vi "SVFA Wrap or Unwrap Phase (XY) (1 Ch).vi"(0 "phase spectrum in":cluster{"X":dbl[], "phase":dbl[]} {"phase" format="%.2f"; "X" format="%.2f"}, 1 "desired wrapping":T8(ring)=enum."Wrap: -180 to 180", 2 "custom wrap range":T1={"minimum phase"=-inf, "maximum phase"=inf}, 4 "spectrum info":T2={"channel name"="", "description"="", "x-axis units"=0, "spectral info"={"spectrum type"=enum."Power [Magnitude^2]", "linear/dB"=enum."linear", "window"=0, "window size"=0, "FFT size"=0}, "engineering units"=1, "custom label"="", "dB reference [EU]"=0.0, "peak units"=enum."rms", "weighting filter"=0, "spectral density?"=FALSE, "unit label"="", "spectrum skewed?"=FALSE, "complimentary spectrum units"=enum."none"} {"x-axis units" items=["Time (s)"=0, "Frequency-CB (Hz)"=1, "Frequency-CPB (Hz)"=1248, "Frequency-Arbitrary (Hz)"=2357, "Quefrency (s)"=2, "Revolutions (rev)"=3, "Order"=4, "Speed (RPM)"=11, "Speed (rad/s)"=21, "Index"=65535]; "weighting filter" items=["Linear", "A-weighting", "B-weighting", "C-weighting", "ITU-R 468-4", "Dolby", "CCITT", "C-message", "Wb", "Wc", "Wd", "We", "Wf", "Wh", "Wj", "Wk", "Wm", "AES17 20 kHz lowpass", "AES17 40 kHz lowpass", "AES17 20 kHz highpass", "AES17 40 kHz highpass"]; "dB reference [EU]" format="%.2f"; "engineering units" items=["custom..."=0, "V"=1, "A"=21, "C"=30, "pC"=31, "s"=32, "-"=29, "Pa"=2, "N"=20, "g"=3, "m/s^2"=4, "m/s"=5, "m"=6, "mm/s"=12, "mm"=13, "micron/s"=14, "micron"=15, "in/s^2"=7, "in/s"=8, "in"=9, "mil/s"=10, "mil"=11, "rad/s^2"=16, "rad/s"=17, "rad"=18, "deg/s^2"=26, "deg/s"=27, "deg"=28, "RPM"=22, "cycle/s^2"=23, "Hz"=24, "cycle"=25, "strain"=19]; "spectral info"."window" items=["None "=0, "Hanning"=1, "Hamming"=2, "Blackman-Harris"=3, "Exact Blackman"=4, "Blackman"=5, "Flat Top"=6, "4 Term B-Harris "=7, "7 Term B-Harris"=8, "Low Sidelobe"=9, "Force - Exponential"=10, "Gaussian"=62]}, 5 "error in (no error)":errorcluster) -> (14 "phase spectrum out":cluster{"X":dbl[], "phase":dbl[]} {"phase" format="%.2f"; "X" format="%.2f"}, 15 "unit label":string, 18 "dup spectrum info":T2={"channel name"="", "description"="", "x-axis units"=0, "spectral info"={"spectrum type"=enum."Power [Magnitude^2]", "linear/dB"=enum."linear", "window"=0, "window size"=0, "FFT size"=0}, "engineering units"=1, "custom label"="", "dB reference [EU]"=0.0, "peak units"=enum."rms", "weighting filter"=0, "spectral density?"=FALSE, "unit label"="", "spectrum skewed?"=FALSE, "complimentary spectrum units"=enum."none"} {"x-axis units" items=["Time (s)"=0, "Frequency-CB (Hz)"=1, "Frequency-CPB (Hz)"=1248, "Frequency-Arbitrary (Hz)"=2357, "Quefrency (s)"=2, "Revolutions (rev)"=3, "Order"=4, "Speed (RPM)"=11, "Speed (rad/s)"=21, "Index"=65535]; "weighting filter" items=["Linear", "A-weighting", "B-weighting", "C-weighting", "ITU-R 468-4", "Dolby", "CCITT", "C-message", "Wb", "Wc", "Wd", "We", "Wf", "Wh", "Wj", "Wk", "Wm", "AES17 20 kHz lowpass", "AES17 40 kHz lowpass", "AES17 20 kHz highpass", "AES17 40 kHz highpass"]; "dB reference [EU]" format="%.2f"; "engineering units" items=["custom..."=0, "V"=1, "A"=21, "C"=30, "pC"=31, "s"=32, "-"=29, "Pa"=2, "N"=20, "g"=3, "m/s^2"=4, "m/s"=5, "m"=6, "mm/s"=12, "mm"=13, "micron/s"=14, "micron"=15, "in/s^2"=7, "in/s"=8, "in"=9, "mil/s"=10, "mil"=11, "rad/s^2"=16, "rad/s"=17, "rad"=18, "deg/s^2"=26, "deg/s"=27, "deg"=28, "RPM"=22, "cycle/s^2"=23, "Hz"=24, "cycle"=25, "strain"=19]; "spectral info"."window" items=["None "=0, "Hanning"=1, "Hamming"=2, "Blackman-Harris"=3, "Exact Blackman"=4, "Blackman"=5, "Flat Top"=6, "4 Term B-Harris "=7, "7 Term B-Harris"=8, "Low Sidelobe"=9, "Force - Exponential"=10, "Gaussian"=62]}, 19 "error out":errorcluster)   [LabVIEW 2017]
doc: "Wraps the phase spectra to the specified range, so that all phase values are coerced to the specified band. You also can use this VI to unwrap phase spectra to eliminate discontinuities with absolute values exceeding 180 degrees = pi radians = 0.5 cycles. Wire data to the <B>phase spectrum in</B> input to determine the polymorphic instance to use or manually select the instance."
uses:
  <vilib>/addons/_NISVFA/_Shared subVIs/Controls/svc_Spectrum Info.ctl
  <vilib>/addons/_NISVFA/_Shared subVIs/Controls/svc_X-Axis Units.ctl
  <vilib>/addons/_NISVFA/_Shared subVIs/Controls/svc_Spectrum Type.ctl
  <vilib>/addons/_NISVFA/_Shared subVIs/Controls/svc_Engineering Units Text Ring.ctl
  <vilib>/addons/_NISVFA/_Shared subVIs/Controls/svc_Weighting Filter Text Ring.ctl
  <vilib>/addons/_NISVFA/_Shared subVIs/Controls/svc_Complimentary Spectrum Units.ctl
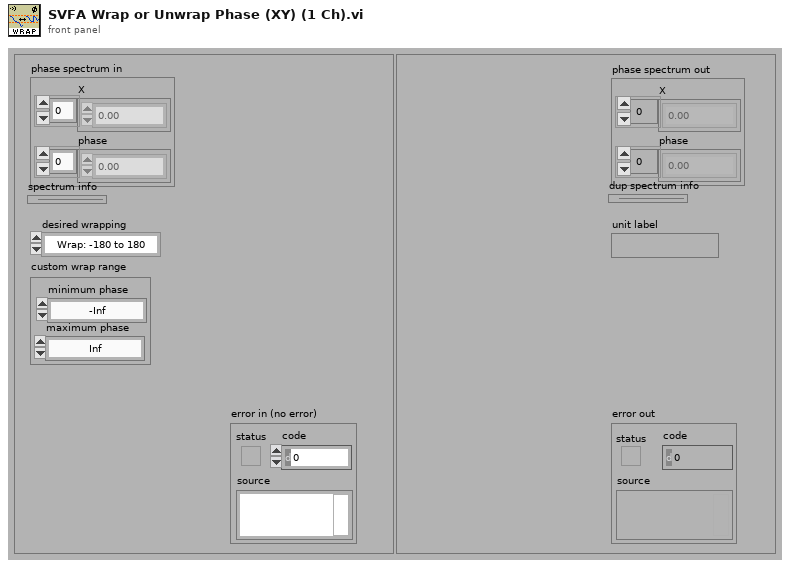
[diagram p1: front panel]
types:
  T1 = cluster{"minimum phase":dbl, "maximum phase":dbl}
  T2 = typedef "svc_Spectrum Info.ctl" = cluster{"channel name":string, "description":string, "x-axis units":T3, "spectral info":cluster{"spectrum type":T4, "linear/dB":enum16{"linear", "dB"}, "window":u16, "window size":i32, "FFT size":i32}, "engineering units":T5, "custom label":string, "dB reference [EU]":dbl, "peak units":enum16{"rms", "peak", "peak-peak"}, "weighting filter":T6, "spectral density?":bool, "unit label":string, "spectrum skewed?":bool, "complimentary spectrum units":T7}
  T3 = typedef "svc_X-Axis Units.ctl" = u16
  T4 = typedef "svc_Spectrum Type.ctl" = enum16{"FFT Spectrum [complex]", "Amplitude [Magnitude]", "Power [Magnitude^2]", "Cross Spectrum [complex]", "Frequency Response [Complex]"}
  T5 = typedef "svc_Engineering Units Text Ring.ctl" = u16
  T6 = typedef "svc_Weighting Filter Text Ring.ctl" = u16
  T7 = typedef "svc_Complimentary Spectrum Units.ctl" = enum16{"none", "radians", "degrees", "cycles", "imaginary"}
  T8 = enum16{"No change", "Unwrap", "Wrap: -360 to 0", "Wrap: -270 to 90", "Wrap: -180 to 180", "Wrap: -90 to 270", "Wrap: 0 to 360", "Wrap: custom range"}
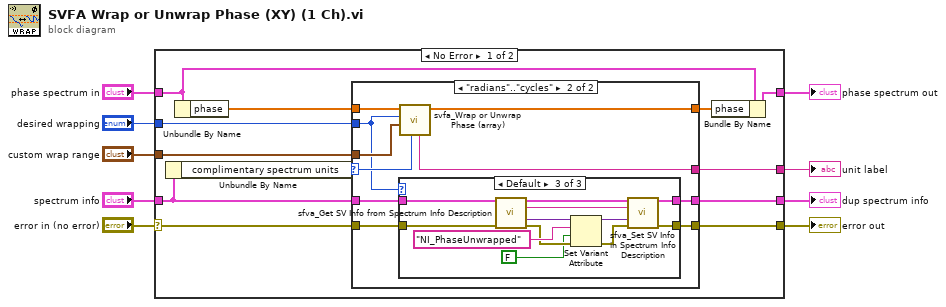
[diagram p0: block diagram]
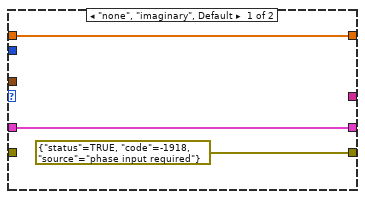
[diagram p2: hidden frame]
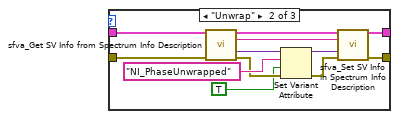
[diagram p4: hidden frame]
diagram:
  n1 = case shown="No Error" "error in (no error)" {
    selector: "error in (no error)" -> [w13 w62]
    tunnel: "phase spectrum in" -> [w16 w63]
    tunnel: [w15 w63] -> w8
    tunnel: [w12 w62] -> w2
    tunnel: "desired wrapping" -> [w18 _]
    tunnel: "spectrum info" -> [w11 w61]
    tunnel: [w10 w61] -> w3
    tunnel: [w19 _] -> w4
    tunnel: "custom wrap range" -> [w17 _]
    frame No Error {
      n2 = Unbundle By Name(w11) -> ("complimentary spectrum units"=w14:T7)
      n3 = Unbundle By Name(w16) -> ("phase"=w20:dbl[])
      n4 = case shown="\"radians\"..\"cycles\"" w14 {
        selector: w14 -> [_ w30]
        tunnel: [w24 w34] -> w21
        tunnel: w20 -> [w24 w33]
        tunnel: [_ w32] -> w19
        tunnel: w18 -> [_ w25]
        tunnel: w17 -> [_ w31]
        tunnel: w13 -> [_ w26]
        tunnel: [errorcluster {"status"=TRUE, "code"=-1918, "source"="phase input required"} ("error IO") w27] -> w12
        tunnel: w11 -> [w22 w29]
        tunnel: [w22 w28] -> w10
        frame "none", "imaginary", Default {
        }
        frame "radians".."cycles" {
          n5 = case shown="Default" w25 {
            tunnel: w29 -> [w36 w41 w53]
            tunnel: [w36 w40 w52] -> w28
            tunnel: [w35 w39 w51] -> w27
            tunnel: w26 -> [w35 w38 w50]
            frame "No change" {
            }
            frame "Unwrap" {
              n6 = call <vilib>:"sfva_Get SV Info from Spectrum Info Description.vi"("spectrum info"=w41, "error in (no error)"=w38) -> ("spectrum info"=w48:T2, "description"=w47:string, "SV Info"=w43:variant, "error out"=w42:errorcluster)  [unwired: 9 in, 1 out]
              n7 = Set Variant Attribute(Variant=w43, name="NI_PhaseUnwrapped", value=TRUE ("replaced"), error in=w42) -> (Variant out=w44:variant, error out=w45:errorcluster)  [unwired: 1 out]
              n8 = call <vilib>:"sfva_Set SV Info in Spectrum Info Description.vi"("spectrum info"=w48, "description"=w47, "SV Info"=w44, "error in (no error)"=w45) -> ("spectrum info"=w40:T2, "error out"=w39:errorcluster)  [unwired: 10 in]
            }
            frame Default {
              n9 = call <vilib>:"sfva_Get SV Info from Spectrum Info Description.vi"("spectrum info"=w53, "error in (no error)"=w50) -> ("spectrum info"=w60:T2, "description"=w59:string, "SV Info"=w55:variant, "error out"=w54:errorcluster)  [unwired: 9 in, 1 out]
              n10 = Set Variant Attribute(Variant=w55, name="NI_PhaseUnwrapped", value=FALSE ("replaced"), error in=w54) -> (Variant out=w56:variant, error out=w57:errorcluster)  [unwired: 1 out]
              n11 = call <vilib>:"sfva_Set SV Info in Spectrum Info Description.vi"("spectrum info"=w60, "description"=w59, "SV Info"=w56, "error in (no error)"=w57) -> ("spectrum info"=w52:T2, "error out"=w51:errorcluster)  [unwired: 10 in]
            }
          }
          n12 = call <vilib>:"svfa_Wrap or Unwrap Phase (array).vi"("phase units"=w30, "custom wrap range"=w31, "desired wrapping"=w25, "phase in"=w33) -> ("phase out"=w34:dbl[], "unit label"=w32:string)  [unwired: 6 in]
        }
      }
      n13 = Bundle By Name(cluster=w16, "phase"=w21) -> (w15:cluster{"X":dbl[], "phase":dbl[]})
    }
    frame Error {
    }
  }
  "phase spectrum out" <- w8
  "error out" <- w2
  "dup spectrum info" <- w3
  "unit label" <- w4
